vi "rqcAlice SPI.SyncDetector Values.vi"(8 "error in":errorcluster, 9 "Comparator level":dbl=1.15 format="%#_13g", 10 "Offset":dbl=1.15 format="%#_13g", 11 "Alice FPGA Reference In":refnum<k20>) -> (0 "error out":errorcluster, 3 "Alice FPGA Reference Out":refnum<k20>)   [LabVIEW 2018]
uses:
  SPI.SubVIs/SPI.SubSystem.ctl
  <vilib>/Utility/error.llb/Error Cluster From Error Code.vi
  <vilib>/rvi/errors/niLvFpgaAdjustHostInterfaceError.vi
  <vilib>/rvi/interface/nirviReadWriteControl/nirviReadWriteControl.xnode
  NiFpgaLv.dll
  <vilib>/rvi/interface/Simulation/niFpgaSimulationCallBeginRW.vi
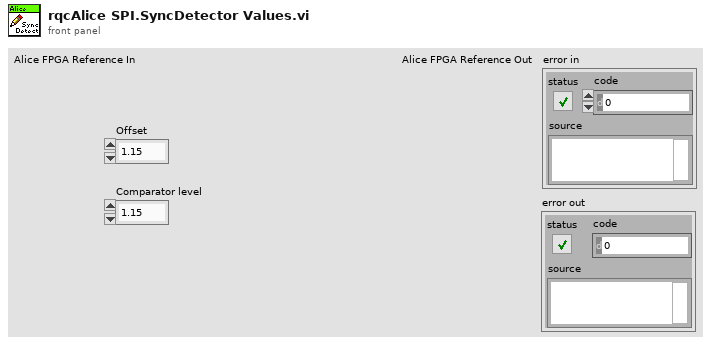
[diagram p1: front panel]
types:
  T1 = typedef "SPI.SubSystem.ctl" = enum8{"N/A", "DelayLine.MSB", "DelayLine.LSB", "Attenuation.dB", "Attenuation.DAC value", "SyncDetector.Offset", "SyncDetector.Comparator"}
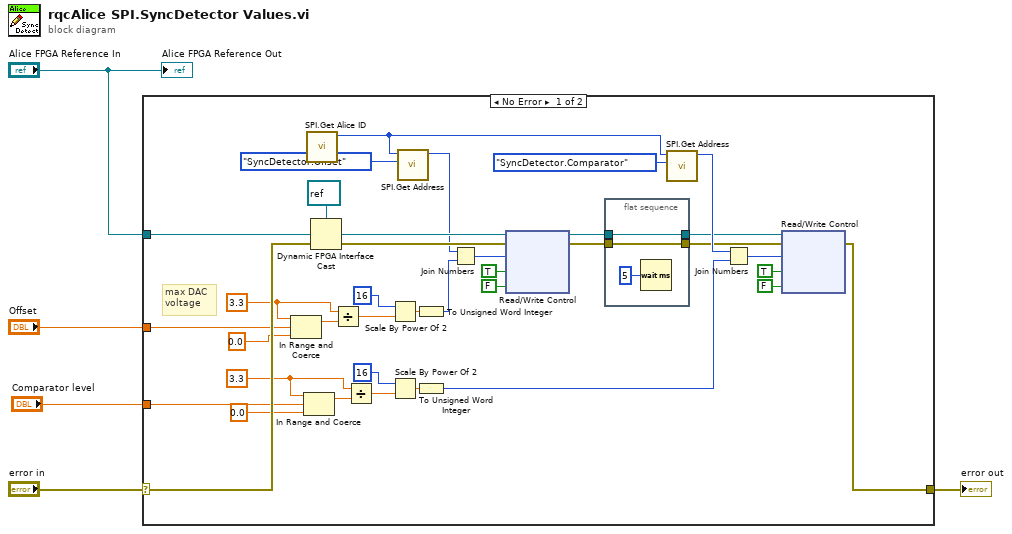
[diagram p0: block diagram]
diagram:
  n1 = case shown="No Error" "error in" {
    selector: "error in" -> [w35 w45]
    tunnel: [w30 w45] -> w4
    tunnel: "Alice FPGA Reference In" -> [w41 _]
    tunnel: "Offset" -> [w25 _]
    tunnel: "Comparator level" -> [w11 _]
    frame No Error {
      w14 = 3.3 ("upper limit")
      w22 = 3.3 ("upper limit")
      # "max DAC\nvoltage"
      n2 = In Range and Coerce(upper limit=w22, x=w25, lower limit=0.0) -> (coerced(x)=w23:dbl)  [unwired: 1 out]
      n3 = In Range and Coerce(upper limit=w14, x=w11, lower limit=0.0) -> (coerced(x)=w13:dbl)  [unwired: 1 out]
      n4 = call "SPI.Get Alice ID.vi"() -> ("Alice.ID"=w29:u8)  [unwired: 11 in]
      n5 = Dynamic FPGA Interface Cast(Session In=refnum<k20> refnum ("Type"), Type=w41) -> (Session Out=w36:refnum<k20>)
      n6 = Divide(x=w22, y=w23) -> (x/y=w21:dbl)
      n7 = Divide(x=w14, y=w13) -> (x/y=w15:dbl)
      n8 = Scale By Power Of 2(n=i16 16, x=w21) -> (x*2^n=w19:dbl)
      n9 = Scale By Power Of 2(n=i16 16, x=w15) -> (x*2^n=w17:dbl)
      n10 = call "SPI.Get Address.vi"("SPI.subSystem"=SPI.SubSystem."SyncDetector.Offset", "ID"=w29) -> ("Address"=w34:u16)  [unwired: 9 in]
      n11 = To Unsigned Word Integer(number=w19) -> (unsigned 16bit integer=w18:u16)
      n12 = To Unsigned Word Integer(number=w17) -> (unsigned 16bit integer=w10:u16)
      n13 = Join Numbers(hi=w34, lo=w18) -> ((hi.lo)=w37:u32)
      n14 = xnode "Read/Write Control"("FPGA VI Reference In"=w36, "error in"=w35, "SPI.data"=w37, "SPI.write"=TRUE ("reset"), "SPI.write"=FALSE ("reset")) -> ("FPGA VI Reference Out"=w9:refnum<k20>, "error out"=w8:errorcluster)
      n15 = flat-sequence {
        tunnel: w9 -> [w43]
        tunnel: [w44] -> w7
        tunnel: w8 -> [w44]
        tunnel: [w43] -> w6
        frame #0 {
          n16 = Wait (ms)(milliseconds to wait=u32 5) -> ()  [unwired: 1 out]
        }
      }
      n17 = call "SPI.Get Address.vi"("SPI.subSystem"=SPI.SubSystem."SyncDetector.Comparator", "ID"=w29) -> ("Address"=w27:u16)  [unwired: 9 in]
      n18 = Join Numbers(hi=w27, lo=w10) -> ((hi.lo)=w26:u32)
      n19 = xnode "Read/Write Control"("FPGA VI Reference In"=w6, "error in"=w7, "SPI.data"=w26, "SPI.write"=TRUE ("reset"), "SPI.write"=FALSE ("reset")) -> ("error out"=w30:errorcluster)  [unwired: 1 out]
    }
    frame Error {
    }
  }
  "error out" <- w4
  "Alice FPGA Reference Out" <- "Alice FPGA Reference In"
